vi "New SinglePlotPanel.vi"(8 "error in (no error)":errorcluster, 9 "Multiplot inputs":T1, 10 "Init options":T2={"UI visible?"=FALSE, "Update rate (ms)"=250, "visible sidebar?"=TRUE, "time to plot (init)"=600.0, "time to plot (max)"=inf, "config file start path"=path ""} {"time to plot (init)" format="%<%H:%M:%S>t"}, 11 "BluePlotHandle":refnum<class "BluePlotHandle.lvclass">) -> (0 "error out":errorcluster, 3 "SinglePlotPanel out":refnum<class "SinglePlotPanel.lvclass">)   [LabVIEW 2021, in "MultiBluePlot.lvlib" / "SinglePlotPanel.lvclass"]
uses:
  SinglePlotPanel.lvclass
  <userlib>/Blue Origin/BluePlot (Open Source)/Classes/BluePlotHandle/BluePlotHandle.lvclass
  <userlib>/Blue Origin/BluePlot (Open Source)/Classes/BluePlotHandle/SubVIs/Init Options.ctl
  SinglePlotPanel.lvclass/SinglePlotPanel.ctl
  <userlib>/Blue Origin/BluePlot (Open Source)/TypeDefs/BlueMultiPlot Inputs.ctl
  <userlib>/Blue Origin/BluePlot (Open Source)/BluePlot.lvlib
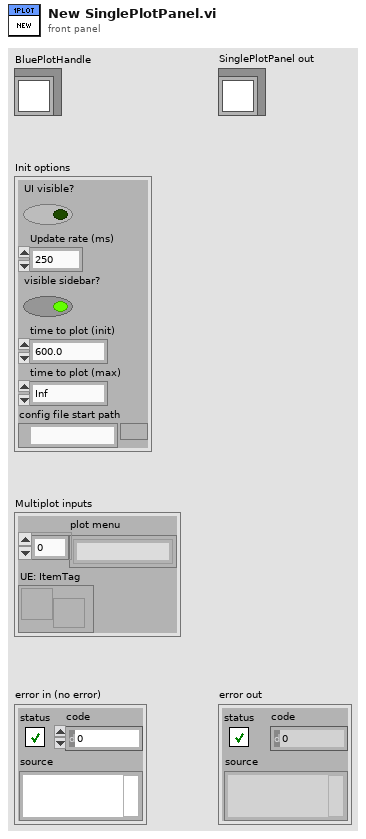
[diagram p1: front panel]
types:
  T1 = typedef "BluePlot.lvlib/BlueMultiPlot Inputs.ctl" = cluster{"plot menu":string[], "UE: ItemTag":refnum<user-event>}
  T2 = typedef "BluePlot.lvlib/BluePlotHandle.lvclass/Init Options.ctl" = cluster{"UI visible?":bool, "Update rate (ms)":u32, "visible sidebar?":bool, "time to plot (init)":dbl, "time to plot (max)":dbl, "config file start path":path}
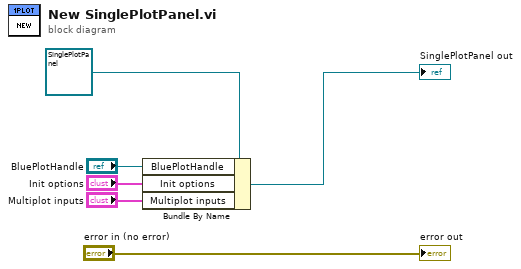
[diagram p0: block diagram]
diagram:
  n1 = Bundle By Name(cluster=refnum<class "SinglePlotPanel.lvclass"> refnum ("SinglePlotPanel out"), "BluePlotHandle"="BluePlotHandle", "Init options"="Init options", "Multiplot inputs"="Multiplot inputs") -> (→"SinglePlotPanel out":refnum<class "SinglePlotPanel.lvclass">)
  "error out" <- "error in (no error)"
